vi "sv_UFF58 Set Function Name.vi"(0 "ID lines (1-3) in":T1, 5 "channel name":string) -> (4 "ID lines (1-3) out":T1, 6 "function name":string)   [LabVIEW 2017, in "SoundVib_UFF58.lvlib"]
doc: "This VI sets the name of the function in the <B>ID lines (1-3) out</B>. If <B>ID lines (1-3) in</B> contains a description, it uses that description for the function. If the description in the <B>ID lines (1-3) in</B> is empty, it uses the value in the <B>channel name</B>. If both the strings are empty, then NONE is sent to <B>function name</B>. It could happen that the name in the <B>ID lines (1-3) out</B> is empty and that is OK."
uses:
  <vilib>/addons/Sound and Vibration/svt_UFF58/SoundVib_UFF58.lvlib
  <vilib>/addons/Sound and Vibration/svt_UFF58/subVIs/sv_IDLines123.ctl
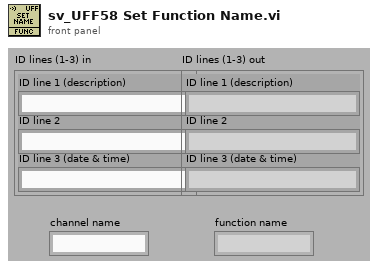
[diagram p1: front panel]
types:
  T1 = typedef "SoundVib_UFF58.lvlib/sv_IDLines123.ctl" = cluster{"ID line 1 (description)":string, "ID line 2":string, "ID line 3 (date & time)":string}
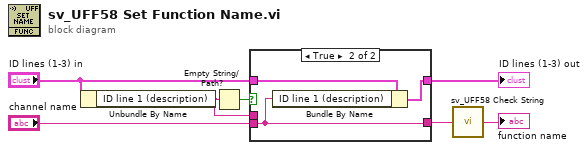
[diagram p0: block diagram]
diagram:
  n1 = Unbundle By Name("ID lines (1-3) in") -> ("ID line 1 (description)"=w7:string)
  n2 = Empty String/Path?(string/path=w7) -> (empty?=w5:bool)
  n3 = case shown="True" w5 {
    tunnel: "ID lines (1-3) in" -> [w9 w12]
    tunnel: "channel name" -> [_ w10]
    tunnel: [w9 w11] -> w4
    tunnel: [w8 w10] -> w2
    tunnel: w7 -> [w8 _]
    frame False {
    }
    frame True {
      n4 = Bundle By Name(cluster=w12, "ID line 1 (description)"=w10) -> (w11:T1)
    }
  }
  "ID lines (1-3) out" <- w4
  n5 = call <vilib>:"sv_UFF58 Check String.vi"("field value"=w2) -> ("output string"=→"function name":string)  [unwired: 13 in, 1 out]
